vi "All Test.vi"() -> ()   [LabVIEW 2020, in "TEST JKI State Machine API.lvlib"]
uses:
  TEST JKI State Machine API.lvlib
panel:
  in  "error in (no error)":errorcluster
  out "error out":errorcluster
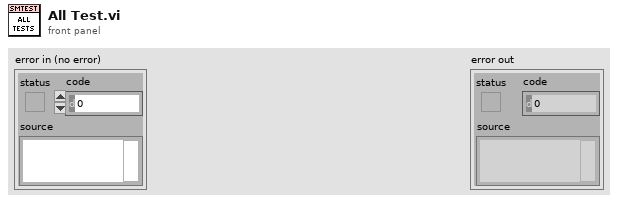
[diagram p1: front panel]
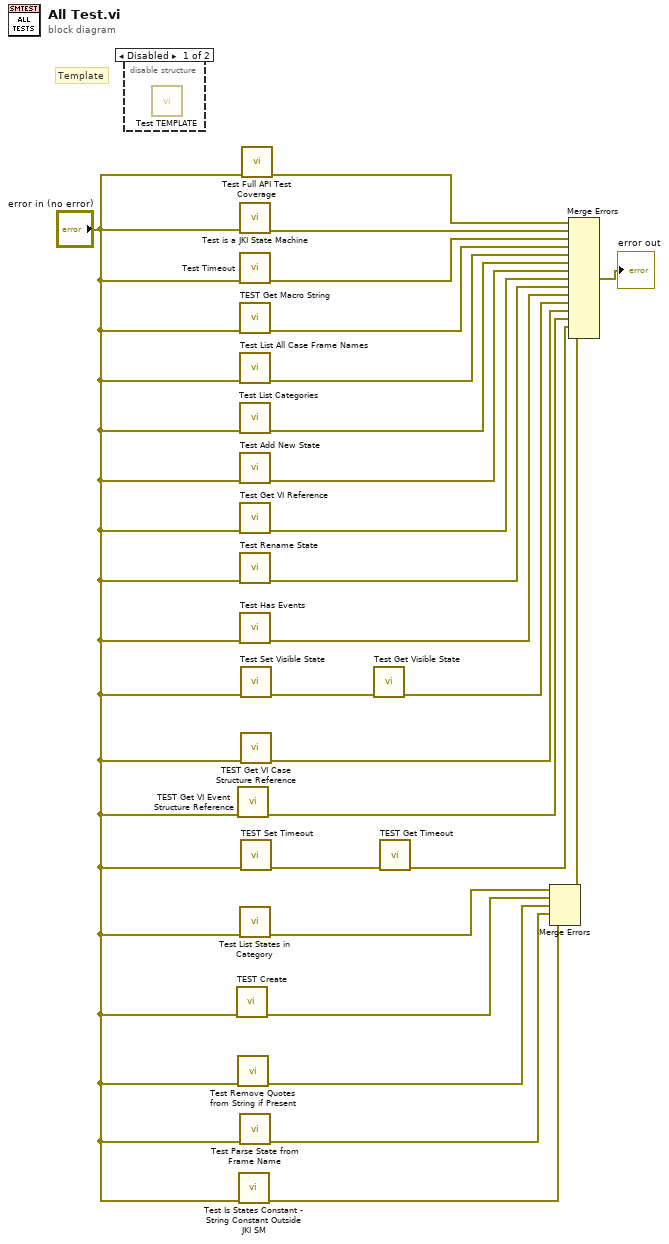
[diagram p0: block diagram]
diagram:
  # "Template"
  n1 = disable-structure shown="Disabled" {
    frame Disabled {
      n2 = call "Test TEMPLATE.vi"() -> ()  [unwired: 11 in, 1 out]
    }
    frame Enabled {
    }
  }
  n3 = call "TEST Create.vi"("error in (no error)"="error in (no error)") -> ("error out"=w5:errorcluster)  [unwired: 10 in]
  n4 = call "TEST Get VI Event Structure Reference.vi"("error in (no error)"="error in (no error)") -> ("error out"=w11:errorcluster)  [unwired: 10 in]
  n5 = call "Test Remove Quotes from String if Present.vi"("error in (no error)"="error in (no error)") -> ("error out"=w4:errorcluster)  [unwired: 10 in]
  n6 = call "Test Is States Constant - String Constant Outside JKI SM.vi"("error in (no error)"="error in (no error)") -> ("error out"=w1:errorcluster)  [unwired: 10 in]
  n7 = call "Test is a JKI State Machine.vi"("error in (no error)"="error in (no error)") -> ("error out"=w23:errorcluster)  [unwired: 10 in]
  n8 = call "Test Timeout.vi"("error in (no error)"="error in (no error)") -> ("error out"=w22:errorcluster)  [unwired: 10 in]
  n9 = call "TEST Get Macro String.vi"("error in (no error)"="error in (no error)") -> ("error out"=w21:errorcluster)  [unwired: 10 in]
  n10 = call "Test List All Case Frame Names.vi"("error in (no error)"="error in (no error)") -> ("error out"=w20:errorcluster)  [unwired: 10 in]
  n11 = call "Test List Categories.vi"("error in (no error)"="error in (no error)") -> ("error out"=w19:errorcluster)  [unwired: 10 in]
  n12 = call "Test Add New State.vi"("error in (no error)"="error in (no error)") -> ("error out"=w18:errorcluster)  [unwired: 10 in]
  n13 = call "Test Get VI Reference.vi"("error in (no error)"="error in (no error)") -> ("error out"=w17:errorcluster)  [unwired: 10 in]
  n14 = call "Test Rename State.vi"("error in (no error)"="error in (no error)") -> ("error out"=w16:errorcluster)  [unwired: 10 in]
  n15 = call "Test Has Events.vi"("error in (no error)"="error in (no error)") -> ("error out"=w15:errorcluster)  [unwired: 10 in]
  n16 = call "Test List States in Category.vi"("error in (no error)"="error in (no error)") -> ("error out"=w7:errorcluster)  [unwired: 10 in]
  n17 = call "Test Parse State from Frame Name.vi"("error in (no error)"="error in (no error)") -> ("error out"=w3:errorcluster)  [unwired: 10 in]
  n18 = call "Test Set Visible State.vi"("error in (no error)"="error in (no error)") -> ("error out"=w13:errorcluster)  [unwired: 10 in]
  n19 = call "TEST Get VI Case Structure Reference.vi"("error in (no error)"="error in (no error)") -> ("error out"=w10:errorcluster)  [unwired: 10 in]
  n20 = call "TEST Set Timeout.vi"("error in (no error)"="error in (no error)") -> ("error out"=w9:errorcluster)  [unwired: 10 in]
  n21 = call "Test Full API Test Coverage.vi"("error in (no error)"="error in (no error)") -> ("error out"=w14:errorcluster)  [unwired: 10 in]
  n22 = call "Test Get Visible State.vi"("error in (no error)"=w13) -> ("error out"=w12:errorcluster)  [unwired: 10 in]
  n23 = call "TEST Get Timeout.vi"("error in (no error)"=w9) -> ("error out"=w8:errorcluster)  [unwired: 10 in]
  n24 = Merge Errors(w7, w5, w4, w3, w1) -> (w6:errorcluster)
  n25 = Merge Errors(w14, w23, w22, w21, w20, w19, w18, w17, w16, w15, w12, w10, w11, w8, w6) -> (→"error out":errorcluster)
